vi "TestExternalDisplay-1.vi"() -> ()   [LabVIEW 2020]
panel:
  in  "Conversion Policy":T1={"Conversion Method"=10, "Minimum Value"=0, "Maximum Value"=0, "# Shifts"=0} {"Conversion Method" items=["Default"=10, "Most Significant Bits"=11, "Full Dynamic"=12, "Downshift"=13, "Given Range"=14, "90% Dynamic"=15, "Given Percent Range"=16]}
  in  "?":bool
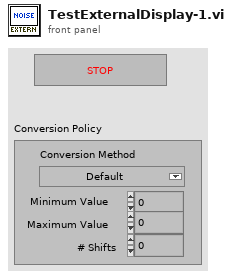
[diagram p1: front panel]
types:
  T1 = cluster{"Conversion Method":u32, "Minimum Value":i32, "Maximum Value":i32, "# Shifts":i32}
  T2 = typedef "Image Type" = u32
  T3 = typedef "IMAQ Image.ctl" = refnum<image>
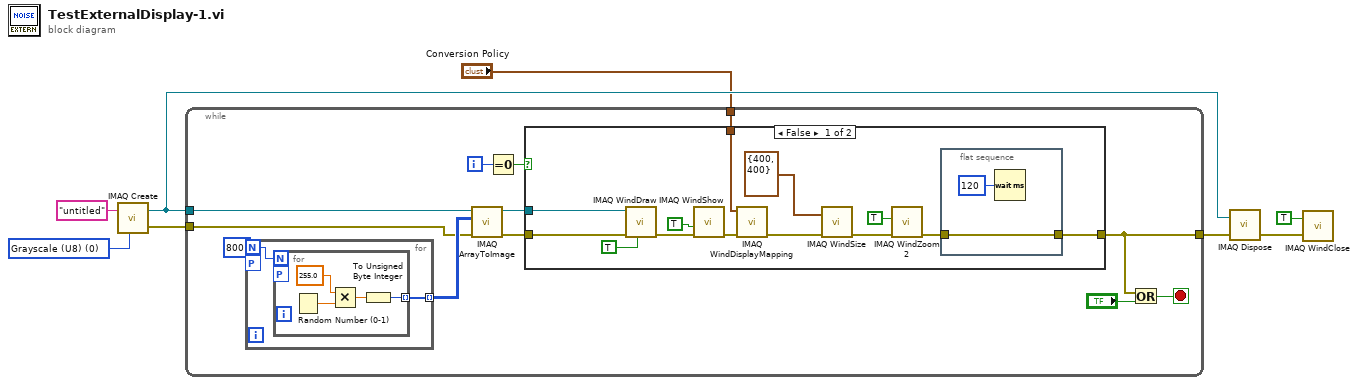
[diagram p0: block diagram]
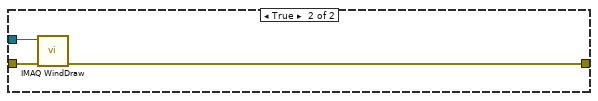
[diagram p2: hidden frame]
diagram:
  w7 = T2 0 items=["Grayscale (U8)", "Grayscale (I16)", "Grayscale (SGL)", "Complex (CSG)", "RGB (U32)", "HSL (U32)", "RGB (U64)", "Grayscale (U16)"] ("Image Type")
  n1 = call "IMAQ Create"("Image Name"="untitled", "Image Type"=w7) -> ("New Image"=w2:T3, "error out"=w6:errorcluster)  [unwired: 3 in]
  n2 = while {
    tunnel: w2 -> [w19]
    tunnel: w6 -> [w13]
    tunnel: [w10] -> w5
    tunnel: "Conversion Policy" -> [w9]
    i -> [w18]
    stop <- w11 stop-if-true
    n3 = for {
      N: 800 -> [w39]
      tunnel: [w40] -> w15 mode=indexing
      workers-P: _ -> [_]
      n4 = for {
        N: w39 -> [_]
        tunnel: [w41] -> w40 mode=indexing
        workers-P: _ -> [_]
        n5 = Random Number (0-1)() -> (number: 0 to 1=w44:dbl)
        n6 = Multiply(x=255.0, y=w44) -> (x*y=w42:dbl)
        n7 = To Unsigned Byte Integer(number=w42) -> (unsigned 8bit integer=w41:u8)
      }
    }
    n8 = call "IMAQ ArrayToImage"("error in (no error)"=w13, "Image Pixels (U8)"=w15, "Image"=w19) -> ("error out"=w14:errorcluster, "Image Out"=w16:T3)  [unwired: 7 in]
    n9 = Equal To 0?(x=w18) -> (x = 0?=w17:bool)
    n10 = case shown="False" w17 {
      tunnel: w16 -> [w32 w38]
      tunnel: w14 -> [w24 w37]
      tunnel: [w22 w36] -> w10
      tunnel: w9 -> [w21 _]
      frame False {
        n11 = call "IMAQ WindDraw"("Resize to Image Size? (Y)"=TRUE, "error in (no error)"=w24, "Image"=w32) -> ("error out"=w33:errorcluster)  [unwired: 7 in, 1 out]
        n12 = call "IMAQ WindShow"("error in (no error)"=w33, "Bring To Front? (N)"=TRUE) -> ("error out"=w30:errorcluster)  [unwired: 4 in, 2 out]
        n13 = call "IMAQ WindDisplayMapping"("error in (no error)"=w30, "Conversion Policy (Default)"=w21) -> ("error out"=w28:errorcluster)  [unwired: 8 in, 1 out]
        n14 = call "IMAQ WindSize"("error in (no error)"=w28, "Width & Height"=cluster{"Width":i32, "Height":i32} {"Width"=400, "Height"=400}) -> ("error out"=w27:errorcluster)  [unwired: 4 in, 2 out]
        n15 = call "IMAQ WindZoom 2"("error in (no error)"=w27, "Zoom to Fit? (False)"=TRUE) -> ("error out"=w23:errorcluster)  [unwired: 6 in, 3 out]
        n16 = flat-sequence {
          tunnel: w23 -> [w34]
          tunnel: [w34] -> w22
          frame #0 {
            n17 = Wait (ms)(milliseconds to wait=u32 120) -> ()  [unwired: 1 out]
          }
        }
      }
      frame True {
        n18 = call "IMAQ WindDraw"("error in (no error)"=w37, "Image"=w38) -> ("error out"=w36:errorcluster)  [unwired: 8 in, 1 out]
      }
    }
    n19 = Or(x=w10, y="?") -> (x .or. y?=w11:bool)
  }
  n20 = call "IMAQ Dispose"("Image"=w2, "error in (no error)"=w5) -> ("error out"=w4:errorcluster)  [unwired: 4 in]
  n21 = call "IMAQ WindClose"("Close All Windows (False)"=TRUE, "error in (no error)"=w4) -> ()  [unwired: 4 in, 1 out]
